vi "Get Thread UI.vi"(8 "error in (no error)":errorcluster, 11 "Component UI in":refnum<class "GE Reflective Memory User Interfaces.lvclass">) -> (0 "error out":errorcluster, 2 "Thread Settings UI":refnum<class "User Interface.lvclass">, 3 "Component UI out":refnum<class "GE Reflective Memory User Interfaces.lvclass">)   [LabVIEW 2017, in "GE Reflective Memory.lvlib" / "GE Reflective Memory User Interfaces.lvclass"]
uses:
  GE Reflective Memory User Interfaces.lvclass
  DSF Core.lvlibp/Classes/User Interface/User Interface.lvclass
  Thread/Thread User Interface.lvclass
  C:/Git/DSF/Components/DSF Core.lvlibp/Classes/User Interface/User Interface.lvclass
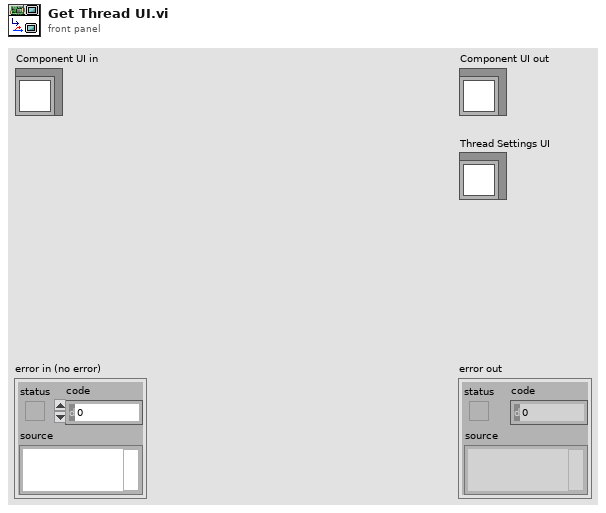
[diagram p1: front panel]
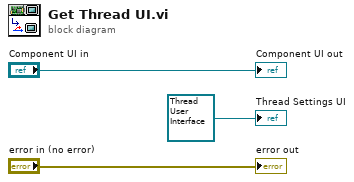
[diagram p0: block diagram]
diagram:
  "error out" <- "error in (no error)"
  "Component UI out" <- "Component UI in"
  "Thread Settings UI" <- refnum<class "Thread User Interface.lvclass"> refnum ("GE Reflective Memory.lvlib:Thread User Interface")
